vi "AFG3352X.set Gauss.vi"(0 "i ref in":refnum<vi>, 2 "Length [us]":dbl, 3 "ms timeout (10000)":i32=10000, 5 "error in (no error)":errorcluster) -> (14 "i ref out":refnum<vi>, 17 "timed out":bool, 19 "error out":errorcluster)   [LabVIEW 2014, in "AFG3352X.lvlib"]
doc: "Top-level part of the Gaussian programming procedure. \n\nHistory: JULY-2004, Stefan Schwarz"
uses:
  AFG3352X.lvlib
  CS_Core/CSApplicationBaseClasses/AFGBase/AFGBase.directionType.ctl
  CS_Core/CSApplicationBaseClasses/AFGBase/AFGBase.serviceType.ctl
  CS_Core/CSApplicationBaseClasses/AFGBase/AFGBase.waveformType.ctl
  CS_Core/CSSystem/CoreDefs/CoreDefs.error_type.ctl
  CS_Core/CSSystem/CoreLib/CoreLib.lvlib
  CS_Core/CSApplicationBaseClasses/AFGBase/AFGBase.lvlib
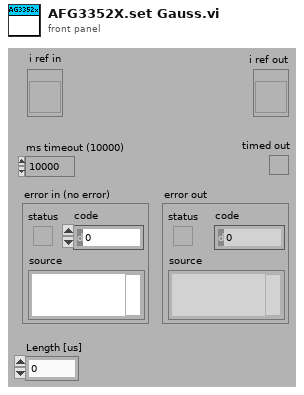
[diagram p1: front panel]
types:
  T1 = typedef "AFGBase.lvlib/AFGBase.waveformType.ctl" = enum16{"sine", "square", "ramp", "pulse", "noise", "DC", "arbitrary", "triangle", "ramp_up", "ramp_down", "amplitude modulation"}
  T2 = typedef "AFGBase.lvlib/AFGBase.serviceType.ctl" = enum16{"frequency", "amplitude", "phase", "DCOffset", "enableOutput", "trigger", "waveformType"}
  T3 = typedef "AFGBase.lvlib/AFGBase.directionType.ctl" = enum16{"unknown", "update actual value", "update nominal value", "update both"}
  T4 = typedef "CoreDefs.error_type.ctl" = enum16{"no error", "can't load process", "can't unload process", "process does not exist", "can't install process", "can't remove process", "unknown function", "time out", "can't execute function", "duplicate queue name", "super not found", "caller queue invalid", "can't ping process", "unknown error", "VISA Error", "VISA timeout", "GPIB timeout", "GPIB error", "communication error", "data type mismatch", "can't read data from OPC server", "can't write data to OPC server", "OET error", "function not implemented", "process already exists", "invalid Shared Variable name", "error writing Shared Variable", "error reading Shared Variable", "invalid client name", "corrupt database", "unknown class", "call not authorized", "parameter out of range", "OET timeout: can't get data to modify", "invalid queue name", "requested operation incompatible with current state", "event undefined", "event disabled", "state undefined", "caller is not a friend", "EventBuilder: bad eventID", "EventBuilder: no DAQ devices", "a thread must not stop itself", "UNUSED ELEMENT4", "DiscArchiver: eventData incomplete", "DiscArchiver: eventData does not belong to run", "DiscArchiver: can't open file", "DiscArchiver: can't write to file", "DiscArchiver: available disc space low", "can't acquire semaphore", "error reading data from database", "notifier object is not existing", "can't register process", "can't unregister process", "illegal event type", "object disabled", "object already exists", "can't change state", "Instrument not found", "no connection to remote node", "invalid reference", "N/A", "UNUSED ELEMENT 1", "element not found", "illegal TCP/IP connection detected", "object does not exist", "invalid access ID", "unknown CS system", "invalid privilige", "unsupported data type", "unsupported server type", "IO server already exists", "Shared Variable already exists"}
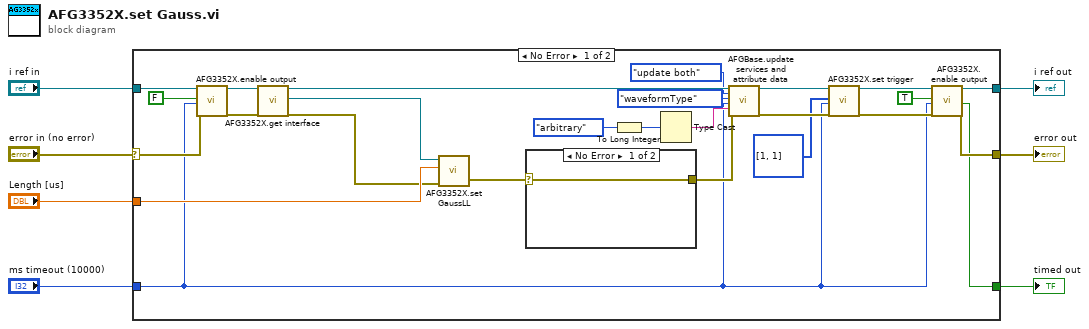
[diagram p0: block diagram]
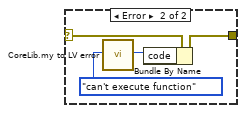
[diagram p2: hidden frame]
diagram:
  n1 = case shown="No Error" "error in (no error)" {
    selector: "error in (no error)" -> [w10 w39]
    tunnel: "i ref in" -> [w11 w40]
    tunnel: "Length [us]" -> [w32 _]
    tunnel: [w31 w40] -> w5
    tunnel: [w30 w39] -> w4
    tunnel: "ms timeout (10000)" -> [w8 _]
    tunnel: [w27 _] -> w2
    frame No Error {
      n2 = call "AFG3352X.enable output.vi"("i ref in"=w11, "outputEnable"=FALSE, "ms timeout (10000)"=w8, "error in (no error)"=w10) -> ("i ref out"=w13:refnum<vi>, "error out"=w12:errorcluster)  [unwired: 13 in, 1 out]
      n3 = call "AFG3352X.get interface.vi"("i ref in"=w13, "error in (no error)"=w12) -> ("i ref out"=w26:refnum<vi>, "interface"=w33:refnum<visa-resource-name>, "error out"=w25:errorcluster)  [unwired: 15 in]
      n4 = call "AFG3352X.set GaussLL.vi"("error in (no error)"=w25, "length [us]"=w32, "VISA in"=w33) -> ("error out"=w29:errorcluster)  [unwired: 1 in, 1 out]
      n5 = case shown="No Error" w29 {
        selector: w29 -> [w34 w38]
        tunnel: [w34 w37] -> w24
        frame No Error {
        }
        frame Error {
          n6 = call "CoreLib.my to LV error.vi"("ErrorTypes"=CoreDefs.error_type."can't execute function") -> ("LV error code"=w36:i32)  [unwired: 17 in, 1 out]
          n7 = Bundle By Name(cluster=w38, "code"=w36) -> (w37:errorcluster)
        }
      }
      n8 = To Long Integer(number=AFGBase.waveformType."arbitrary" ("waveformType")) -> (32bit integer=w19:i32)
      n9 = Type Cast(x=w19) -> (*(type *) &x=w20:string)  [unwired: 1 in]
      n10 = call "AFGBase.update services and attribute data.vi"("i ref in"=w26, "direction"=AFGBase.directionType."update both", "service"=AFGBase.serviceType."waveformType", "ms timeout (10000)"=w8, "value"=w20, "error in (no error)"=w24) -> ("i ref out"=w18:refnum<vi>, "error out"=w17:errorcluster)  [unwired: 11 in, 1 out]
      n11 = call "AFG3352X.set trigger.vi"("i ref in"=w18, "triggerParameters"=i16[] [1, 1], "ms timeout (10000)"=w8, "error in (no error)"=w17) -> ("i ref out"=w15:refnum<vi>, "error out"=w14:errorcluster)  [unwired: 13 in, 1 out]
      n12 = call "AFG3352X.enable output.vi"("i ref in"=w15, "outputEnable"=TRUE, "ms timeout (10000)"=w8, "error in (no error)"=w14) -> ("i ref out"=w31:refnum<vi>, "timed out"=w27:bool, "error out"=w30:errorcluster)  [unwired: 13 in]
    }
    frame Error {
    }
  }
  "error out" <- w4
  "i ref out" <- w5
  "timed out" <- w2
